vi "Configure Channel.vi"(0 "VISA resource name":refnum<visa-resource-name>, 1 "Enable Channel (T: Enable)":bool=TRUE, 2 "Input Impedance (0: 1M ohm)":u16(ring) items=["1M", "75", "50"], 5 "Channel (0: Channel 1)":u16(ring) items=["Channel 1", "Channel 2", "Channel 3", "Channel 4", "Math", "Reference 1", "Reference 2", "Reference 3", "Reference 4", "Bus 1", "Bus 2"], 7 "Vertical Coupling (1: DC)":u16(ring)=1 items=["AC", "DC", "Ground"], 9 "Probe Attenuation (1)":dbl=1.0, 11 "error in (no error)":errorcluster, 12 "Vertical Range (10.0 V)":dbl=10.0, 13 "Vertical Offset (0.0 V)":dbl, 14 "Bandwidth (0: FULL)":u16(ring) items=["FULL", "250 MHz", "150 MHz", "20 MHz"]) -> (4 "VISA resource name out":refnum<visa-resource-name>, 15 "error out":errorcluster)   [LabVIEW 2016, in "Tektronix DPO MSO 2000 4000 Series.lvlib"]
doc: "Enables or disables the selected channel. Configures the vertical properties of the oscilloscope for a specified channel if the channel is enabled. The settings don't take effect if the channel is disabled."
uses:
  Tektronix DPO MSO 2000 4000 Series.lvlib
panel:
  # "Input Channel Parameters"
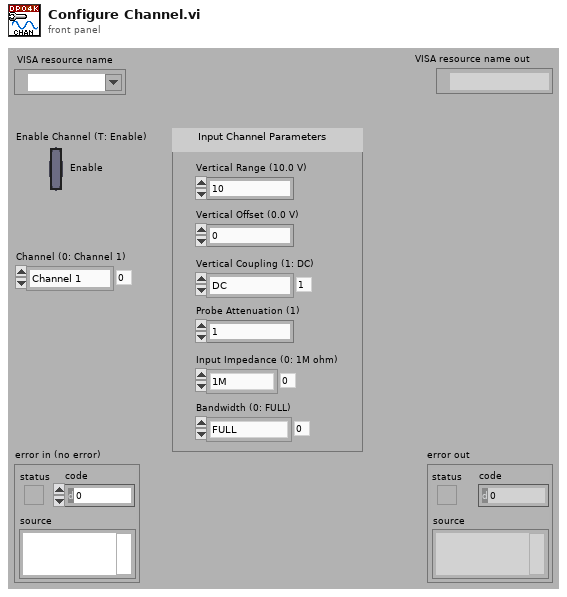
[diagram p1: front panel]
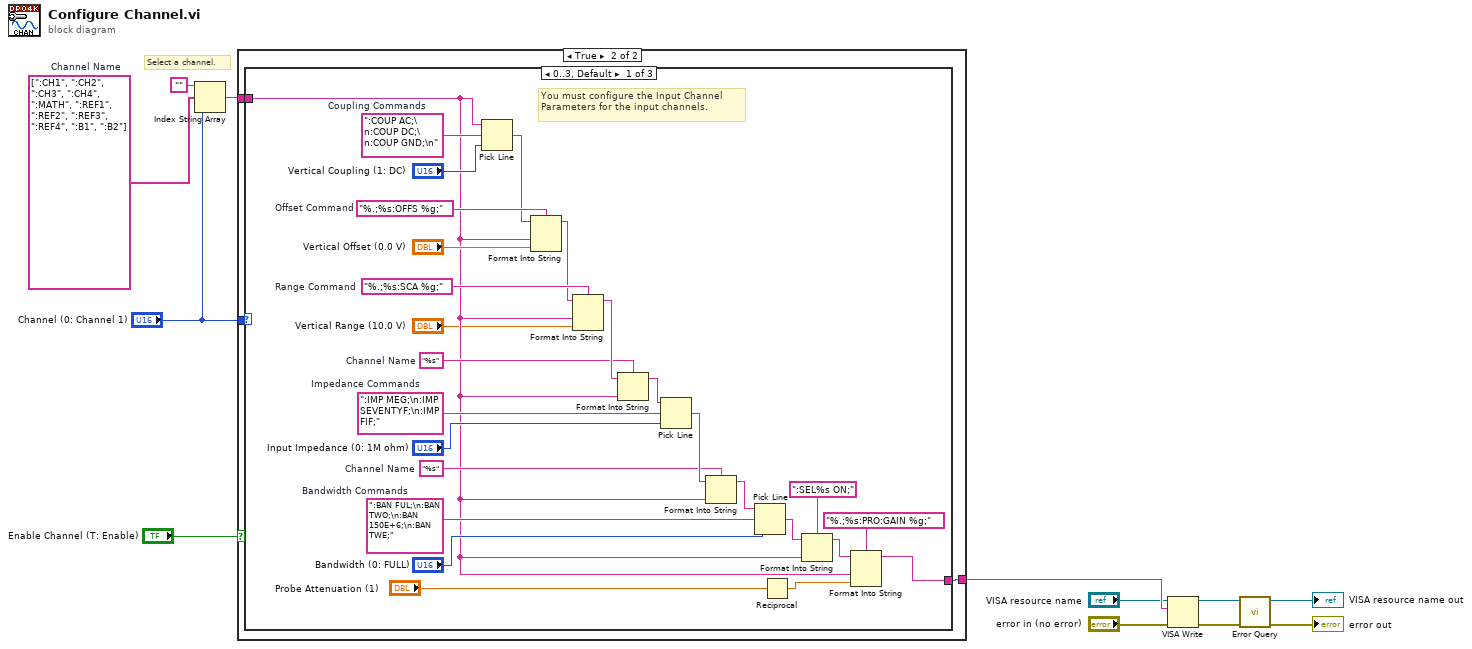
[diagram p0: block diagram]
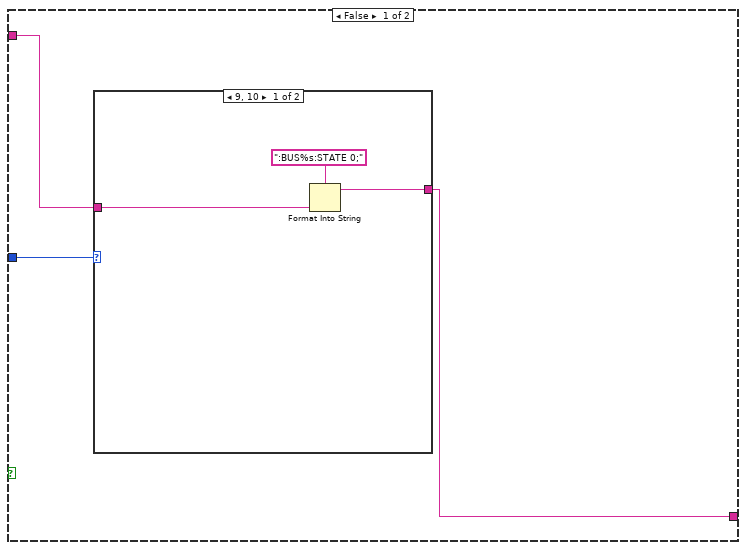
[diagram p2: hidden frame]
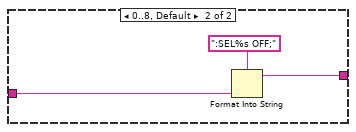
[diagram p3: hidden frame]
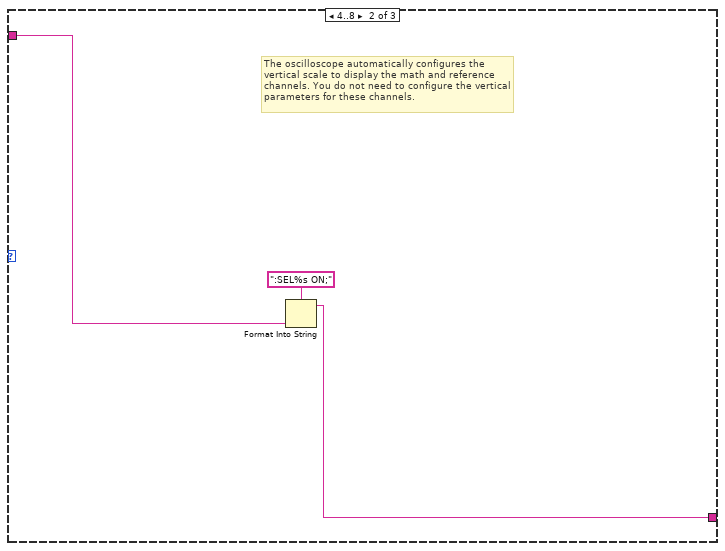
[diagram p4: hidden frame]
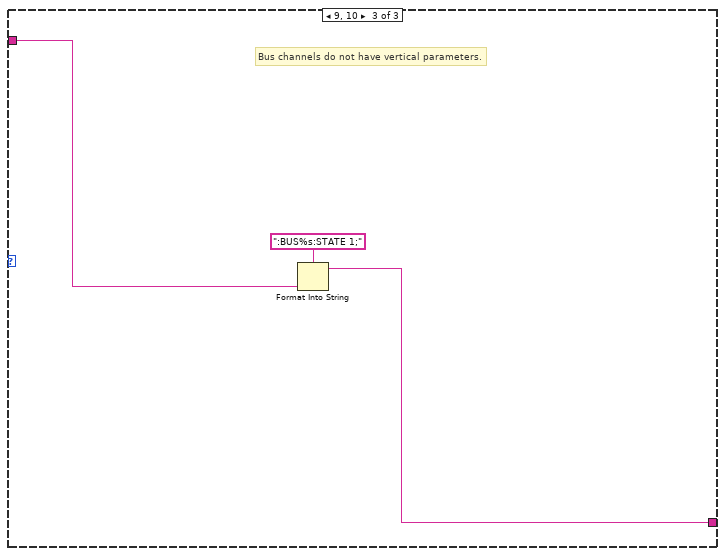
[diagram p5: hidden frame]
diagram:
  w5 = string[] [":CH1", ":CH2", ":CH3", ":CH4", ":MATH", ":REF1", ":REF2", ":REF3", ":REF4", ":B1", ":B2"]  # Channel Name
  # "Select a channel."
  n1 = Index String Array(1:"Channel (0: Channel 1)", 2:w5, 3:"") -> (0:w6:string)
  n2 = case shown="True" "Enable Channel (T: Enable)" {
    tunnel: w6 -> [w14 w23]
    tunnel: "Channel (0: Channel 1)" -> [w15 w24]
    tunnel: [w13 w22] -> w3
    frame False {
      n3 = case shown="9, 10" w15 {
        tunnel: w14 -> [w17 w20]
        tunnel: [w16 w19] -> w13
        frame 9, 10 {
          n4 = Format Into String(format string=":BUS%s:STATE 0;", w17) -> (resulting string=w16:string)  [unwired: 2 in, 1 out]
        }
        frame 0..8, Default {
          n5 = Format Into String(format string=":SEL%s OFF;", w20) -> (resulting string=w19:string)  [unwired: 2 in, 1 out]
        }
      }
    }
    frame True {
      n6 = case shown="0..3, Default" w24 {
        tunnel: w23 -> [w26 w51 w54]
        tunnel: [w29 w52 w55] -> w22
        frame 0..3, Default {
          w35 = ":BAN FUL;\n:BAN TWO;\n:BAN 150E+6;\n:BAN TWE;"  # Bandwidth Commands
          w37 = "%s"  # Channel Name
          w38 = "%s"  # Channel Name
          w40 = ":IMP MEG;\n:IMP SEVENTYF;\n:IMP FIF;"  # Impedance Commands
          w46 = "%.;%s:SCA %g;"  # Range Command
          w48 = "%.;%s:OFFS %g;"  # Offset Command
          w50 = ":COUP AC;\n:COUP DC;\n:COUP GND;\n"  # Coupling Commands
          # "You must configure the Input Channel\nParameters for the input channels."
          n7 = Pick Line(string ("")=w26, multi-line string=w50, line index="Vertical Coupling (1: DC)") -> (output string=w45:string)
          n8 = Format Into String(format string=w48, initial string=w45, w26, "Vertical Offset (0.0 V)") -> (resulting string=w44:string)  [unwired: 1 in, 1 out]
          n9 = Format Into String(format string=w46, initial string=w44, w26, "Vertical Range (10.0 V)") -> (resulting string=w42:string)  [unwired: 1 in, 1 out]
          n10 = Format Into String(format string=w38, initial string=w42, w26) -> (resulting string=w41:string)  [unwired: 1 in, 1 out]
          n11 = Pick Line(string ("")=w41, multi-line string=w40, line index="Input Impedance (0: 1M ohm)") -> (output string=w39:string)
          n12 = Format Into String(format string=w37, initial string=w39, w26) -> (resulting string=w36:string)  [unwired: 1 in, 1 out]
          n13 = Pick Line(string ("")=w36, multi-line string=w35, line index="Bandwidth (0: FULL)") -> (output string=w32:string)
          n14 = Reciprocal(x="Probe Attenuation (1)") -> (1/x=w28:dbl)
          n15 = Format Into String(format string=":SEL%s ON;", initial string=w32, w26) -> (resulting string=w31:string)  [unwired: 1 in, 1 out]
          n16 = Format Into String(format string="%.;%s:PRO:GAIN %g;", initial string=w31, w26, w28) -> (resulting string=w29:string)  [unwired: 1 in, 1 out]
        }
        frame 4..8 {
          # "The oscilloscope automatically configures the vertical scale to display the math and reference channels. You do not need to configure the vertical parameters for these channels."
          n17 = Format Into String(format string=":SEL%s ON;", w51) -> (resulting string=w52:string)  [unwired: 2 in, 1 out]
        }
        frame 9, 10 {
          # "Bus channels do not have vertical parameters."
          n18 = Format Into String(format string=":BUS%s:STATE 1;", w54) -> (resulting string=w55:string)  [unwired: 2 in, 1 out]
        }
      }
    }
  }
  n19 = VISA Write(VISA resource name="VISA resource name", write buffer=w3, error in (no error)="error in (no error)") -> (VISA resource name out=w10:refnum<visa-resource-name>, error out=w9:errorcluster)  [unwired: 1 out]
  n20 = call "Error Query.vi"("error in (no error)"=w9, "VISA resource name"=w10) -> ("error out"=→"error out":errorcluster, "VISA resource name out"=→"VISA resource name out":refnum<visa-resource-name>)  [unwired: 6 in, 2 out]
